vi "readExcel.vi"(1 "xlsx_path":string) -> (0 "JSON":string)   [LabVIEW 2022 SP3]
panel:
  out "error out":errorcluster
  # "например E:/Programming/LabView/readExcel/test.xlsx"
  # "Модуль читает страницу groups и выдает результат в строке формата JSON"
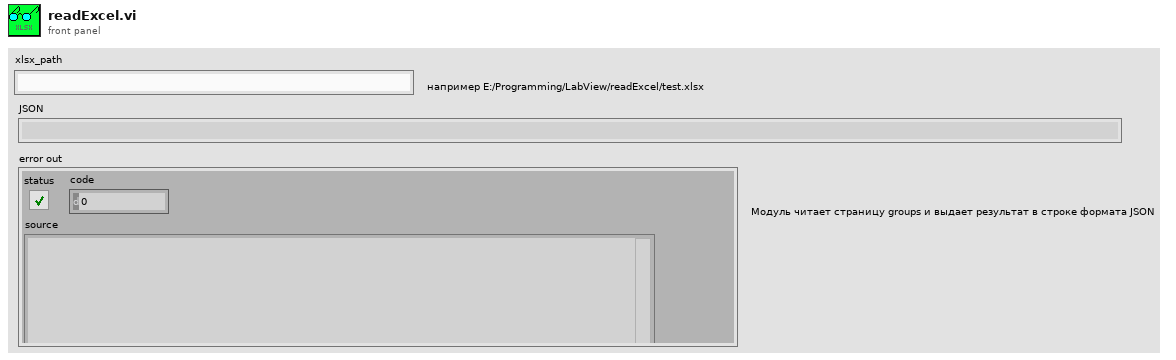
[diagram p1: front panel]
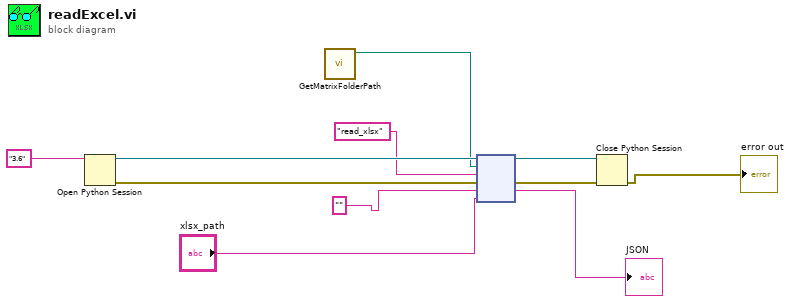
[diagram p0: block diagram]
diagram:
  n1 = Open Python Session(python version="3.6" ("Python version")) -> (session out=w6:refnum<k35>, error out=w7:errorcluster)  [unwired: 2 in]
  n2 = call <vilib>:"GetMatrixFolderPath.vi"() -> ("module path"=w1:path)  [unwired: 11 in]
  n3 = node(w6, w1, "read_xlsx" ("function name"), w7, "", "xlsx_path") -> (w10:refnum<k35>, w9:errorcluster, →"JSON":string)  [unwired: 1 in, 2 out]
  n4 = Close Python Session(session in=w10, error in=w9) -> (11:→"error out":errorcluster)
